vi "final (3).vi"() -> ()   [LabVIEW 2020]
uses:
  <vilib>/Instr/_visa.llb/VISA Configure Serial Port (Instr).vi
panel:
  out "RPM":i64(knob) scale=0.0..250.0
  in  "stop":bool
  out "water gate":bool
  in  "PWM LED":i64(knob) scale=0.0..250.0
  in  "NO2":bool
  in  "NO1":bool
  out "water":dbl(slide) scale=0.0..400.0
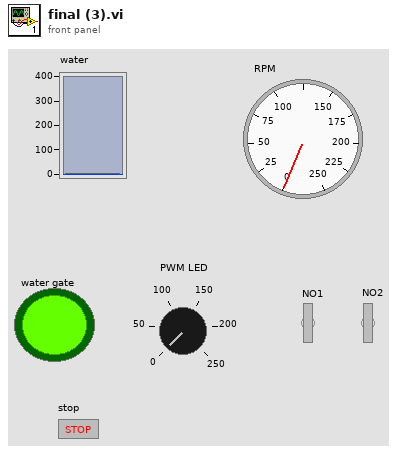
[diagram p1: front panel]
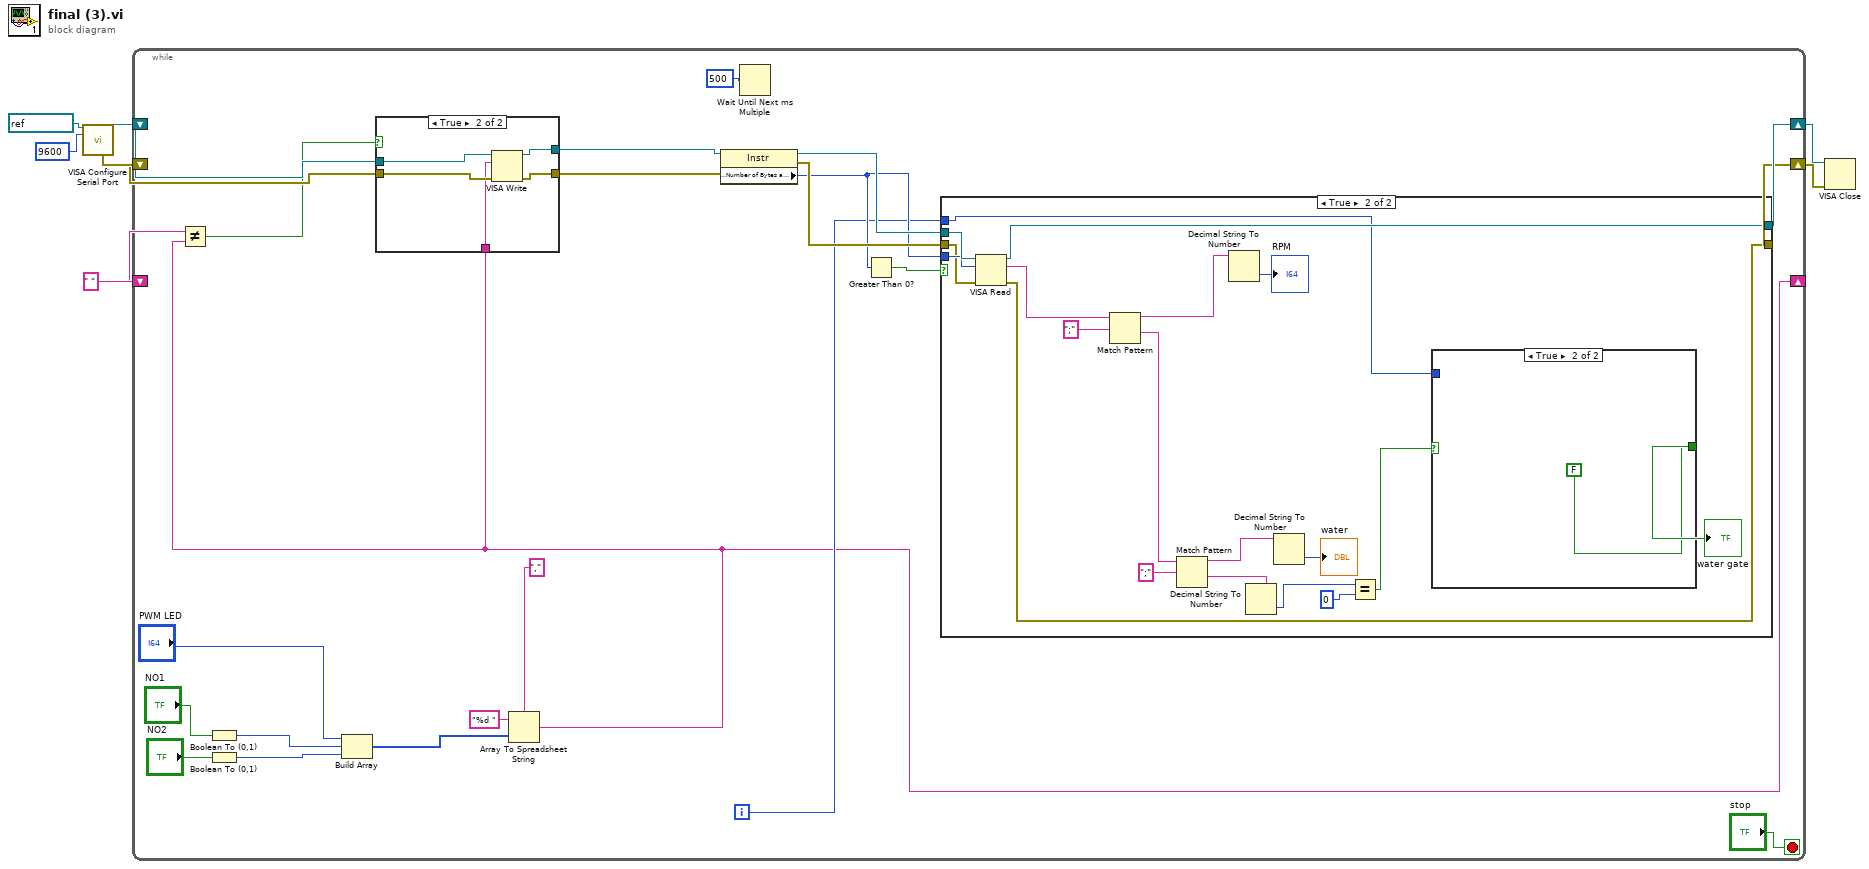
[diagram p0: block diagram]
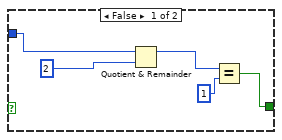
[diagram p3: hidden frame]
diagram:
  n1 = call-poly "VISA Configure Serial Port"("VISA resource name"=refnum<visa-resource-name> "COM3", "baud rate (9600)"=9600) -> ("VISA resource name out"=w7:refnum<visa-resource-name>, "error out"=w6:errorcluster)  [unwired: 12 in]
  n2 = while {
    shift-right: [w22] -> w2
    shift-left: w7 -> [w30]
    shift-right: [w21] -> w1
    shift-left: w6 -> [w29]
    shift-right: [w10] -> _
    shift-left: " " ("spreadsheet string") -> [w11]
    i -> [w20]
    stop <- "stop" stop-if-true
    n3 = Boolean To (0,1)(Boolean="NO1") -> (0, 1=w16:i16)
    n4 = Boolean To (0,1)(Boolean="NO2") -> (0, 1=w15:i16)
    n5 = Build Array("PWM LED", w16, w15) -> (w14:i64[])
    n6 = Array To Spreadsheet String(delimiter (Tab)=",", array=w14, 3:"%d " ("format string")) -> (spreadsheet string=w10:string)
    n7 = Not Equal?(x=w11, y=w10) -> (x != y?=w13:bool)
    n8 = case shown="True" w13 {
      tunnel: w30 -> [w60 w65]
      tunnel: w29 -> [w59 w64]
      tunnel: [w60 w63] -> w28
      tunnel: [w59 w62] -> w27
      tunnel: w10 -> [_ w61]
      frame False {
      }
      frame True {
        n9 = VISA Write(VISA resource name=w65, write buffer=w61, error in (no error)=w64) -> (VISA resource name out=w63:refnum<visa-resource-name>, error out=w62:errorcluster)  [unwired: 1 out]
      }
    }
    n10 = property class="Instr"(reference=w28, error in=w27) -> (reference out=w26:refnum<visa-resource-name>, error out=w25:errorcluster, "Serial Settings:Number of Bytes at Serial Port"=w23:u32)
    n11 = Wait Until Next ms Multiple(millisecond multiple=u32 500) -> ()  [unwired: 1 out]
    n12 = Greater Than 0?(x=w23) -> (x > 0?=w24:bool)
    n13 = case shown="True" w24 {
      tunnel: w26 -> [w33 w52]
      tunnel: w25 -> [w32 w50]
      tunnel: w23 -> [_ w51]
      tunnel: [w33 w49] -> w22
      tunnel: [w32 w48] -> w21
      tunnel: w20 -> [_ w38]
      frame False {
      }
      frame True {
        n14 = VISA Read(VISA resource name=w52, byte count=w51, error in (no error)=w50) -> (VISA resource name out=w49:refnum<visa-resource-name>, read buffer=w47:string, error out=w48:errorcluster)  [unwired: 1 out]
        n15 = Match Pattern(string=w47, regular expression=";") -> (before substring=w46:string, after substring=w35:string)  [unwired: 1 in, 2 out]
        n16 = Match Pattern(string=w35, regular expression=";") -> (before substring=w44:string, after substring=w42:string)  [unwired: 1 in, 2 out]
        n17 = Decimal String To Number(string=w46) -> (number=→"RPM":i32)  [unwired: 2 in, 1 out]
        n18 = Decimal String To Number(string=w42) -> (number=w34:i32)  [unwired: 2 in, 1 out]
        n19 = Decimal String To Number(string=w44) -> (number=→"water":i32)  [unwired: 2 in, 1 out]
        n20 = Equal?(x=w34, y=0) -> (x = y?=w40:bool)
        n21 = case shown="True" w40 {
          tunnel: [w53 FALSE ("water gate")] -> w39
          tunnel: w38 -> [w57 _]
          frame False {
            n22 = Quotient & Remainder(x=w57, y=2) -> (x-y*floor(x/y)=w55:i32)  [unwired: 1 out]
            n23 = Equal?(x=w55, y=1) -> (x = y?=w53:bool)
          }
          frame True {
          }
        }
        "water gate" <- w39
      }
    }
  }
  n24 = VISA Close(VISA resource name=w2, error in (no error)=w1) -> ()  [unwired: 1 out]
